vi "Stay Alive.vi"(8 "error in (no error)":errorcluster, 11 "Animal in":refnum<class "Animal.lvclass">) -> (0 "error out":errorcluster, 3 "Animal out":refnum<class "Animal.lvclass">)   [LabVIEW 2020, in "Animal.lvclass"]
uses:
  Animal.lvclass
  Animal.lvclass/Animal.ctl
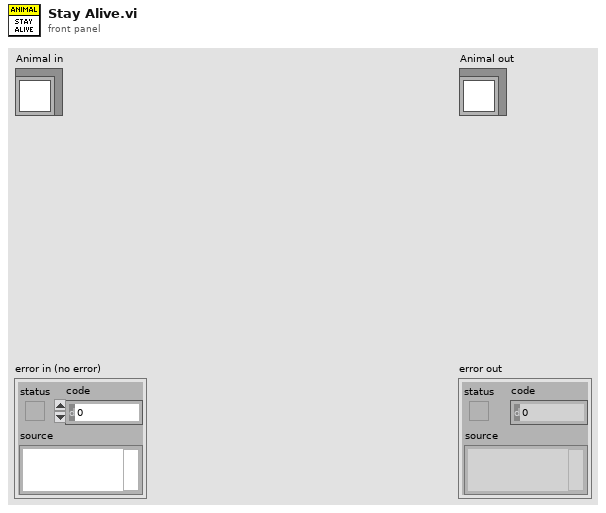
[diagram p1: front panel]
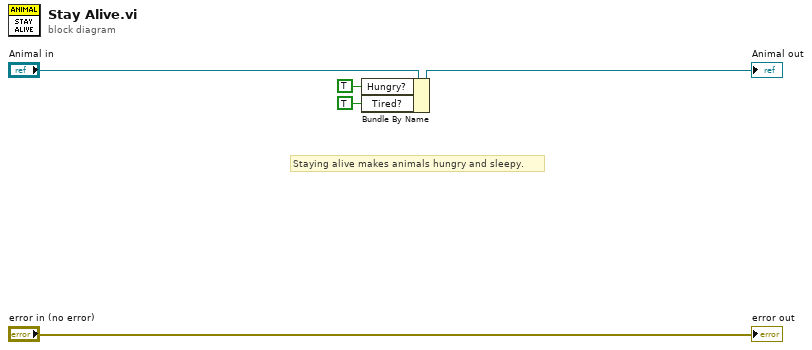
[diagram p0: block diagram]
diagram:
  # "Staying alive makes animals hungry and sleepy."
  n1 = Bundle By Name(cluster="Animal in", "Hungry?"=TRUE, "Tired?"=TRUE) -> (→"Animal out":refnum<class "Animal.lvclass">)
  "error out" <- "error in (no error)"
